vi "Complete_Controller_w_optics - Copy.vi"() -> ()   [LabVIEW 2014]
uses:
  <vilib>/LabVIEW Interface for Arduino/Type Defs/Arduino Resource.ctl
  <vilib>/LabVIEW Interface for Arduino/Type Defs/Board Type.ctl
  <vilib>/Instr/_visa.llb/VISA Configure Serial Port (Instr).vi
  <vilib>/Utility/file.llb/Write To Spreadsheet File (string).vi
  <vilib>/Utility/file.llb/Write To Spreadsheet File (DBL).vi
  <vilib>/Utility/file.llb/Read From Spreadsheet File (string).vi
  <vilib>/DAQmx/read.llb/DAQmx Read (Analog 1D DBL NChan 1Samp).vi
  <vilib>/DAQmx/write.llb/DAQmx Write (Analog 1D DBL NChan 1Samp).vi
  <vilib>/DAQmx/write.llb/DAQmx Write (Digital Bool 1Line 1Point).vi
  Environmental Chamber LabVIEW and Instruments/Drivers and Software/keithley_6430/Keithley 6430/Public/Data/Read (Single Point).vi
  Environmental Chamber LabVIEW and Instruments/Drivers and Software/LabVIEW 8.2 Drivers/keithley_24xx/Keithley 24XX/Public/Data/Read (Single Point).vi
  Environmental Chamber LabVIEW and Instruments/Drivers and Software/keithley_24xx/Keithley 24XX/Keithley 24XX.lvlib
  Environmental Chamber LabVIEW and Instruments/Drivers and Software/keithley_6430/Keithley 6430/Keithley 6430.lvlib
  <vilib>/LabVIEW Interface for Arduino/LabVIEW Interface for Arduino.lvlib
panel:
  out "Currently saving data":bool
  in  "Data saving":T1(radio)
  in  "Integration Time (ms)":i32=80 caption="Inter scan delay ms"
  in  "Optical Smoothing Level":i32 min=0 max=4 step=1
  in  "Number of Scans to Average":i32=1 min=1 max=10000 step=1
  in  "Digitizer Clock Rate Setting":i32=3 min=1 max=3
  out "Critical Error":bool
  in  "Save spectra file path":path=path "C:/Users/User/Desktop/Chamber Data/perovskites/2015-08-04 spectra"
  in  "Aquire spectra":bool
  in  "Seconds between  spectra":dbl caption="Time Target (s)"
  out "Spectrum":cluster{"Wavelengths":dbl[], "buffer out":sgl[]}(graph)
  out "output param":i32
  out "Sequence time left (hrs)":dbl caption="min"
  out "Sequence Preview":cluster{dbl[], dbl[]}[](graph)
  out "Pressure Control 3":bool caption="Pressure Control"
  in  "valve % open":dbl=100.0 min=0.0 max=100.0 step=5.0
  in  "Vapor\nflow\n(sccm)":sgl(slide) min=0 max=100 step=1 scale=0.0..200.0
  out "Actual":dbl
  out "Boolean 3":bool
  out "Actual":dbl
  out "Boolean":bool
  in  "Gas\nflow\n(sccm)":sgl(slide) min=0 max=100 step=1 scale=0.0..200.0
  in  "Desired pressure":dbl min=0.0 max=760.0 step=5.0
  out "Valve position (%)":dbl
  in  "Pressure Control":enum32{"Set % open ", " Set pressure  (Torr)"}(radio)
  out "Pressure Control 2":bool caption="Pressure Control"
  out "Keithley 6430":bool
  out "J-Kem":bool caption="J-Kem Temp"
  out "J-Kem Temp (C)":cluster{dbl}(graph)
  out "Keithley 2420":bool caption="Keithley 2430"
  out "Pressure Control":bool
  out "SRS QCM":bool
  out "MHz":dbl format="%.6f"
  out "Ohm":dbl format="%.4e"
  out "Waveform Chart 7":cluster{dbl, "Resistance out":dbl}(graph)
  out "Chamber Pressure (Torr)":cluster{"f":dbl}(graph)
  in  "Start recording after":dbl caption="min"
  in  "Auto stop after":bool
  in  "hrs":dbl=1000.0 min=0.0
  out "Start Time":string
  out "Elapsed (min)":dbl caption="Elapsed Time (s)"
  in  "Delay between data points (s)":dbl caption="sec" min=0.0 max=30.0 format="%#_13g"
  in  "Turbo pump auto on":bool=TRUE
  in  "stop":bool
  in  "Experiment Notes":string
  in  "Clear all charts":bool
  out "Save data file path":path
  out "Waveform Chart 2":cluster{"f":dbl, "f":dbl}(graph)
  out "Keithley 2420 (Ohm)":cluster{"Resistance":sgl}(graph)
  out "Keithley 6430 (Ohm)":cluster{"Measurement":dbl}(graph)
  in  "Tab Control":T2(tab)
  out "run sequence table":string[][](table) caption="Sequence to run"
  in  "Run Sequence":bool
  out "Current step":i32
  out "Step time remaining (min)":dbl caption="min" format="%#_1g"
  in  "Import sequence file":path
  in  "Use excel file\nfor sequence?":bool
  in  "Pressure Mode":T3(radio)
  in  "User-defined\nsequence":string[][](table) caption="Create sequence"
  in  "Partial pressure of solvent (%)":dbl=100.0 min=0.0 max=100.0 step=5.0
  in  "Arduino":bool
  out "temp\n(C)":string
  out "gas\nsensor":string
  out "Arduino humidity (%)":cluster{dbl}(graph)
  in  "rapidox O2 Sensor":bool
  in  "setnag O2 Pump":bool
  in  "Baud Rate 2":i32(ring)=2 items=["2400", "4800", "9600", "19200", "38400", "57600", "115200"]
  in  "Com Port":i32(ring) items=["Com 1", "Com 2", "Com 3", "Com 4", "Com 5", "Com 6", "COM 7", "COM 8", "COM 9", "COM 10", "COM 11", "COM 12", "com 13", "COM 14"]
  in  "Com Port 2":i32(ring) items=["Com 1", "Com 2", "Com 3", "Com 4", "Com 5", "Com 6", "COM 7", "COM 8", "COM 9", "COM 10", "COM 11", "COM 12", "com 13", "COM 14"]
  out "Torr":dbl
  out "%":dbl
  out "atm":dbl
  out "Waveform Chart":cluster{dbl}(graph)
  out "O2 Concentration (PPM)":dbl
  out "Waveform Chart 6":cluster{dbl}(graph)
  out "Waveform Chart 8":cluster{dbl, "Resistance out":dbl}(graph)
  # "QCM"
  # "Currently Unused"
  # "QCM"
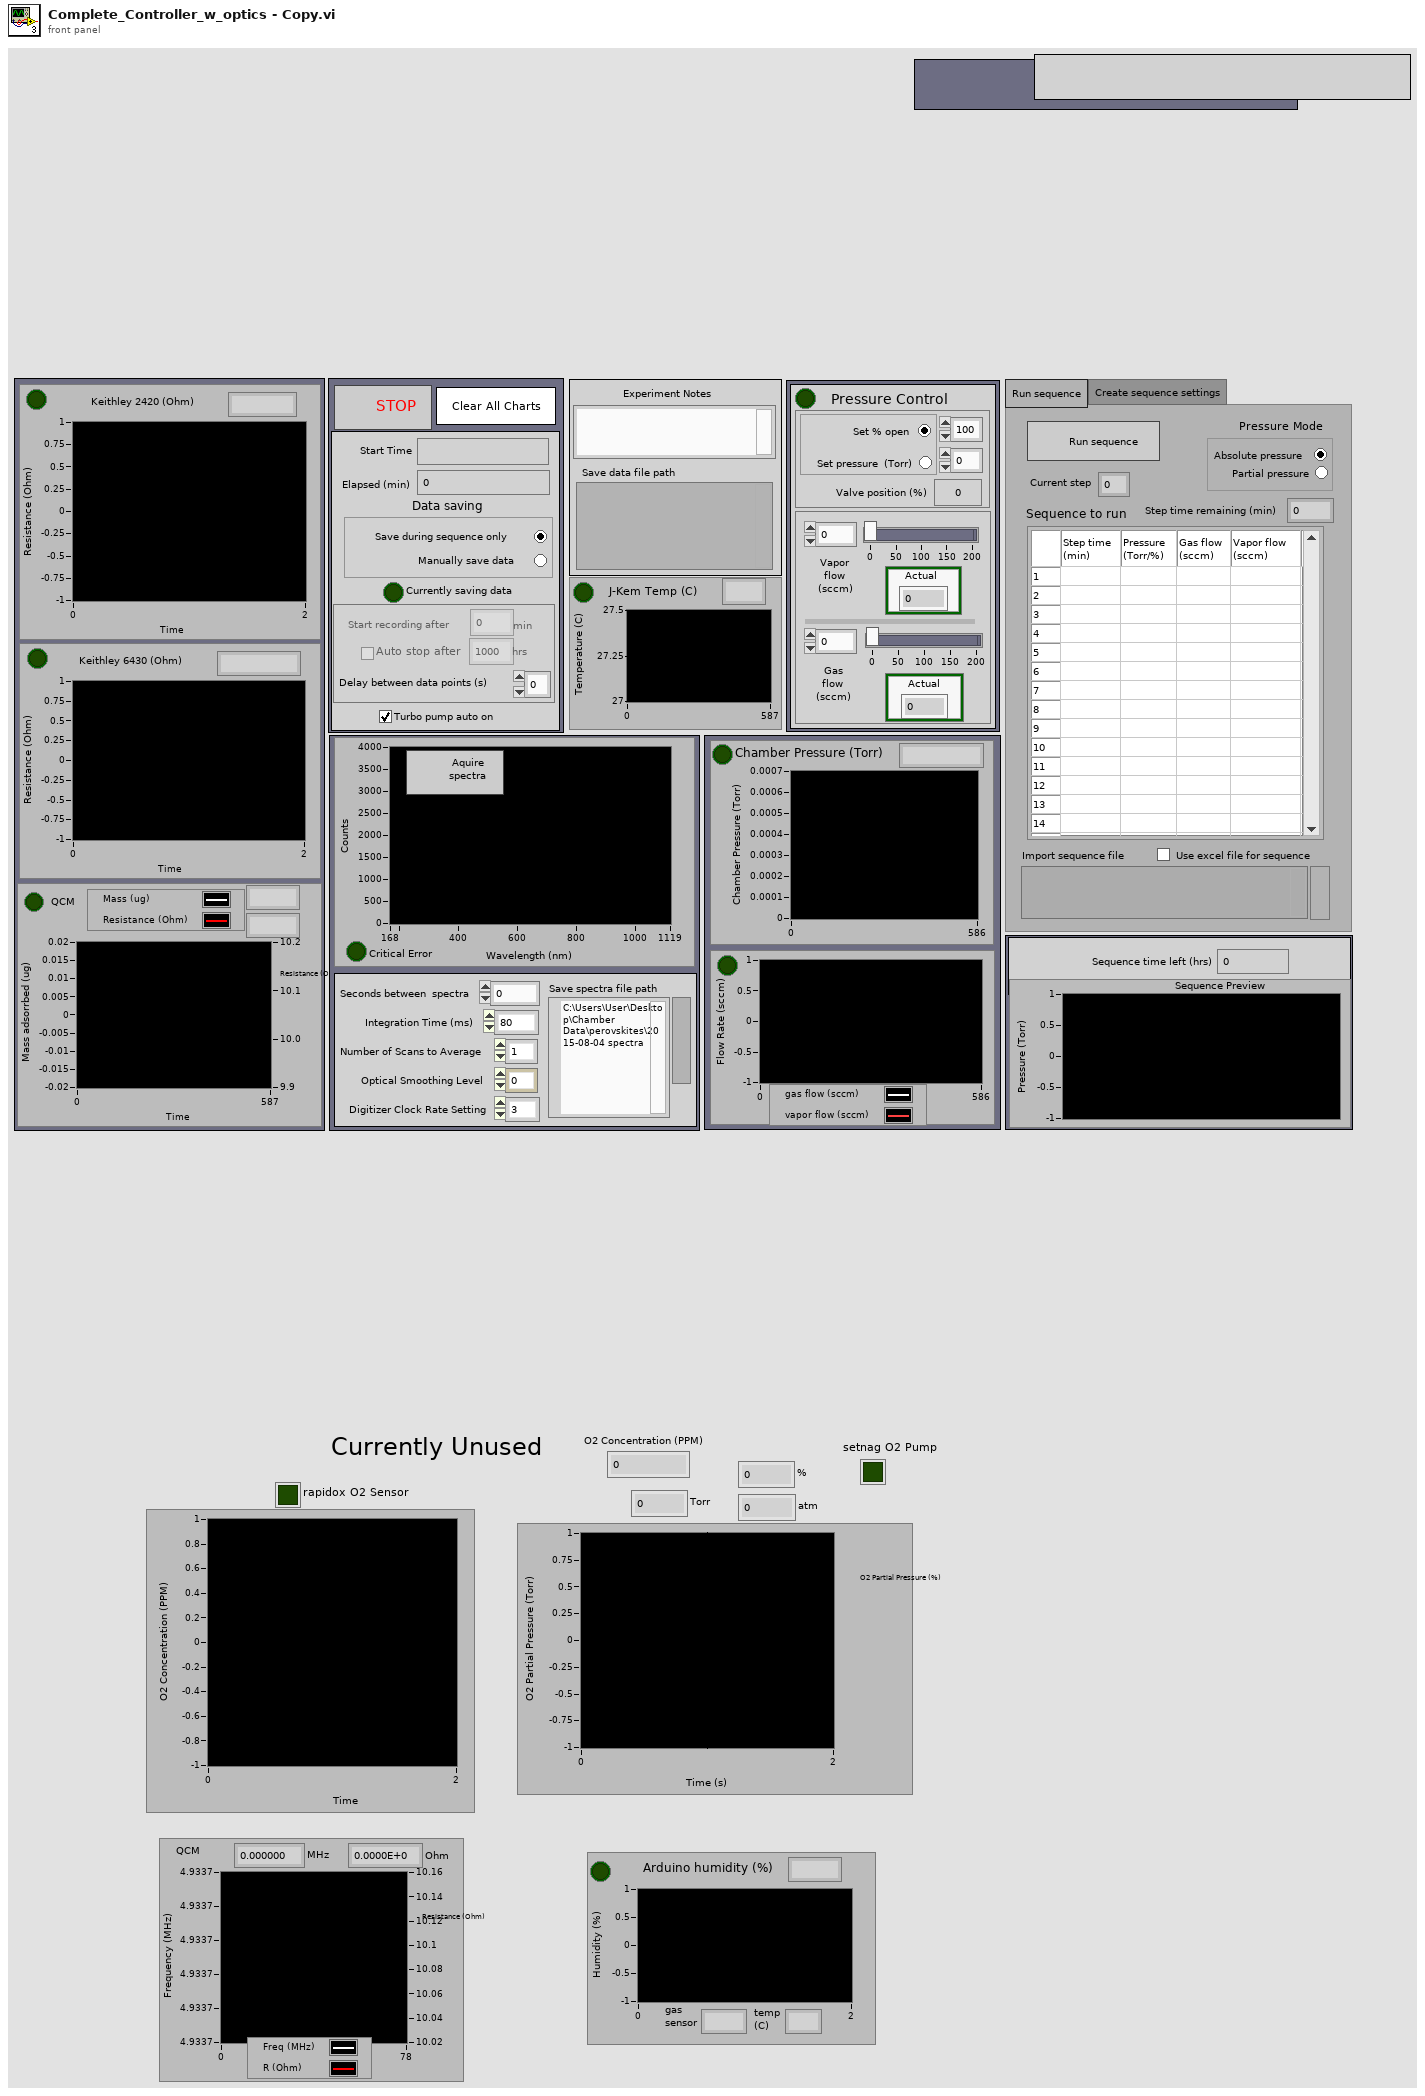
[diagram p1: front panel]
types:
  T1 = enum32{"Save during sequence only", " Manually save data"}
  T2 = enum32{"Run sequence", "Create sequence settings"}
  T3 = enum32{"Absolute pressure ", " Partial pressure"}
  T4 = enum16{"open", "open or create", "create or replace", "create", "open (read only)"}
  T5 = enum16{"no parity", "odd parity", "even parity", "mark parity", "space parity"}
  T6 = cluster{bool, "VISA resource name":refnum<visa-resource-name>, "error out":errorcluster}
  T7 = cluster{bool, "VISA resource name out":refnum<visa-resource-name>, "error out":errorcluster}
  T8 = cluster{"task out":refnum<k21>, "error out":errorcluster, "task out":refnum<k21>, "error out":errorcluster, "task out":refnum<k21>, "error out":errorcluster, "VISA resource name":refnum<visa-resource-name>, "error out":errorcluster}
  T9 = cluster{"task out":refnum<k21>, "error out":errorcluster, "task out":refnum<k21>, "error out":errorcluster, "task out":refnum<k21>, "error out":errorcluster, "VISA resource name out":refnum<visa-resource-name>, "error out":errorcluster}
  T10 = cluster{"Coefficients":ext[], "Wavelengths":dbl[]}[]
  T11 = cluster{"Integration Time (ms)":i32, "Number of Scans to Average":i32, "Optical Smoothing Level":i32, "Digitizer Clock Rate Setting":i32, "Temp  Compensation ":bool}[]
  T12 = cluster{"Integration Time (ms)":i32, "Number of Scans to Average":i32, "Optical Smoothing Level":i32, "Digitizer Clock Rate Setting":i32, "Temp  Compensation ":bool}
  T13 = cluster{"Coefficients":ext[], "Wavelengths":dbl[]}
  T14 = cluster{bool, "VISA out":refnum<visa-resource-name>, "error out":errorcluster}
  T15 = cluster{"Boolean":bool, "VISA resource name out":refnum<visa-resource-name>, "error out":errorcluster}
  T16 = enum8{"Enabled", "Disabled", "Disabled and Grayed Out"}
  T17 = typedef "LabVIEW Interface for Arduino.lvlib/Arduino Resource.ctl" = cluster{"VISA resource":refnum<visa-resource-name>, "Board Type":T18, "Connection Type":enum8{"USB / Serial"}, "Bytes Per Packet (15)":u8}
  T18 = typedef "LabVIEW Interface for Arduino.lvlib/Board Type.ctl" = enum16{"Uno", "Dimuelanove w/Atmega 328", "Mega 2560"}
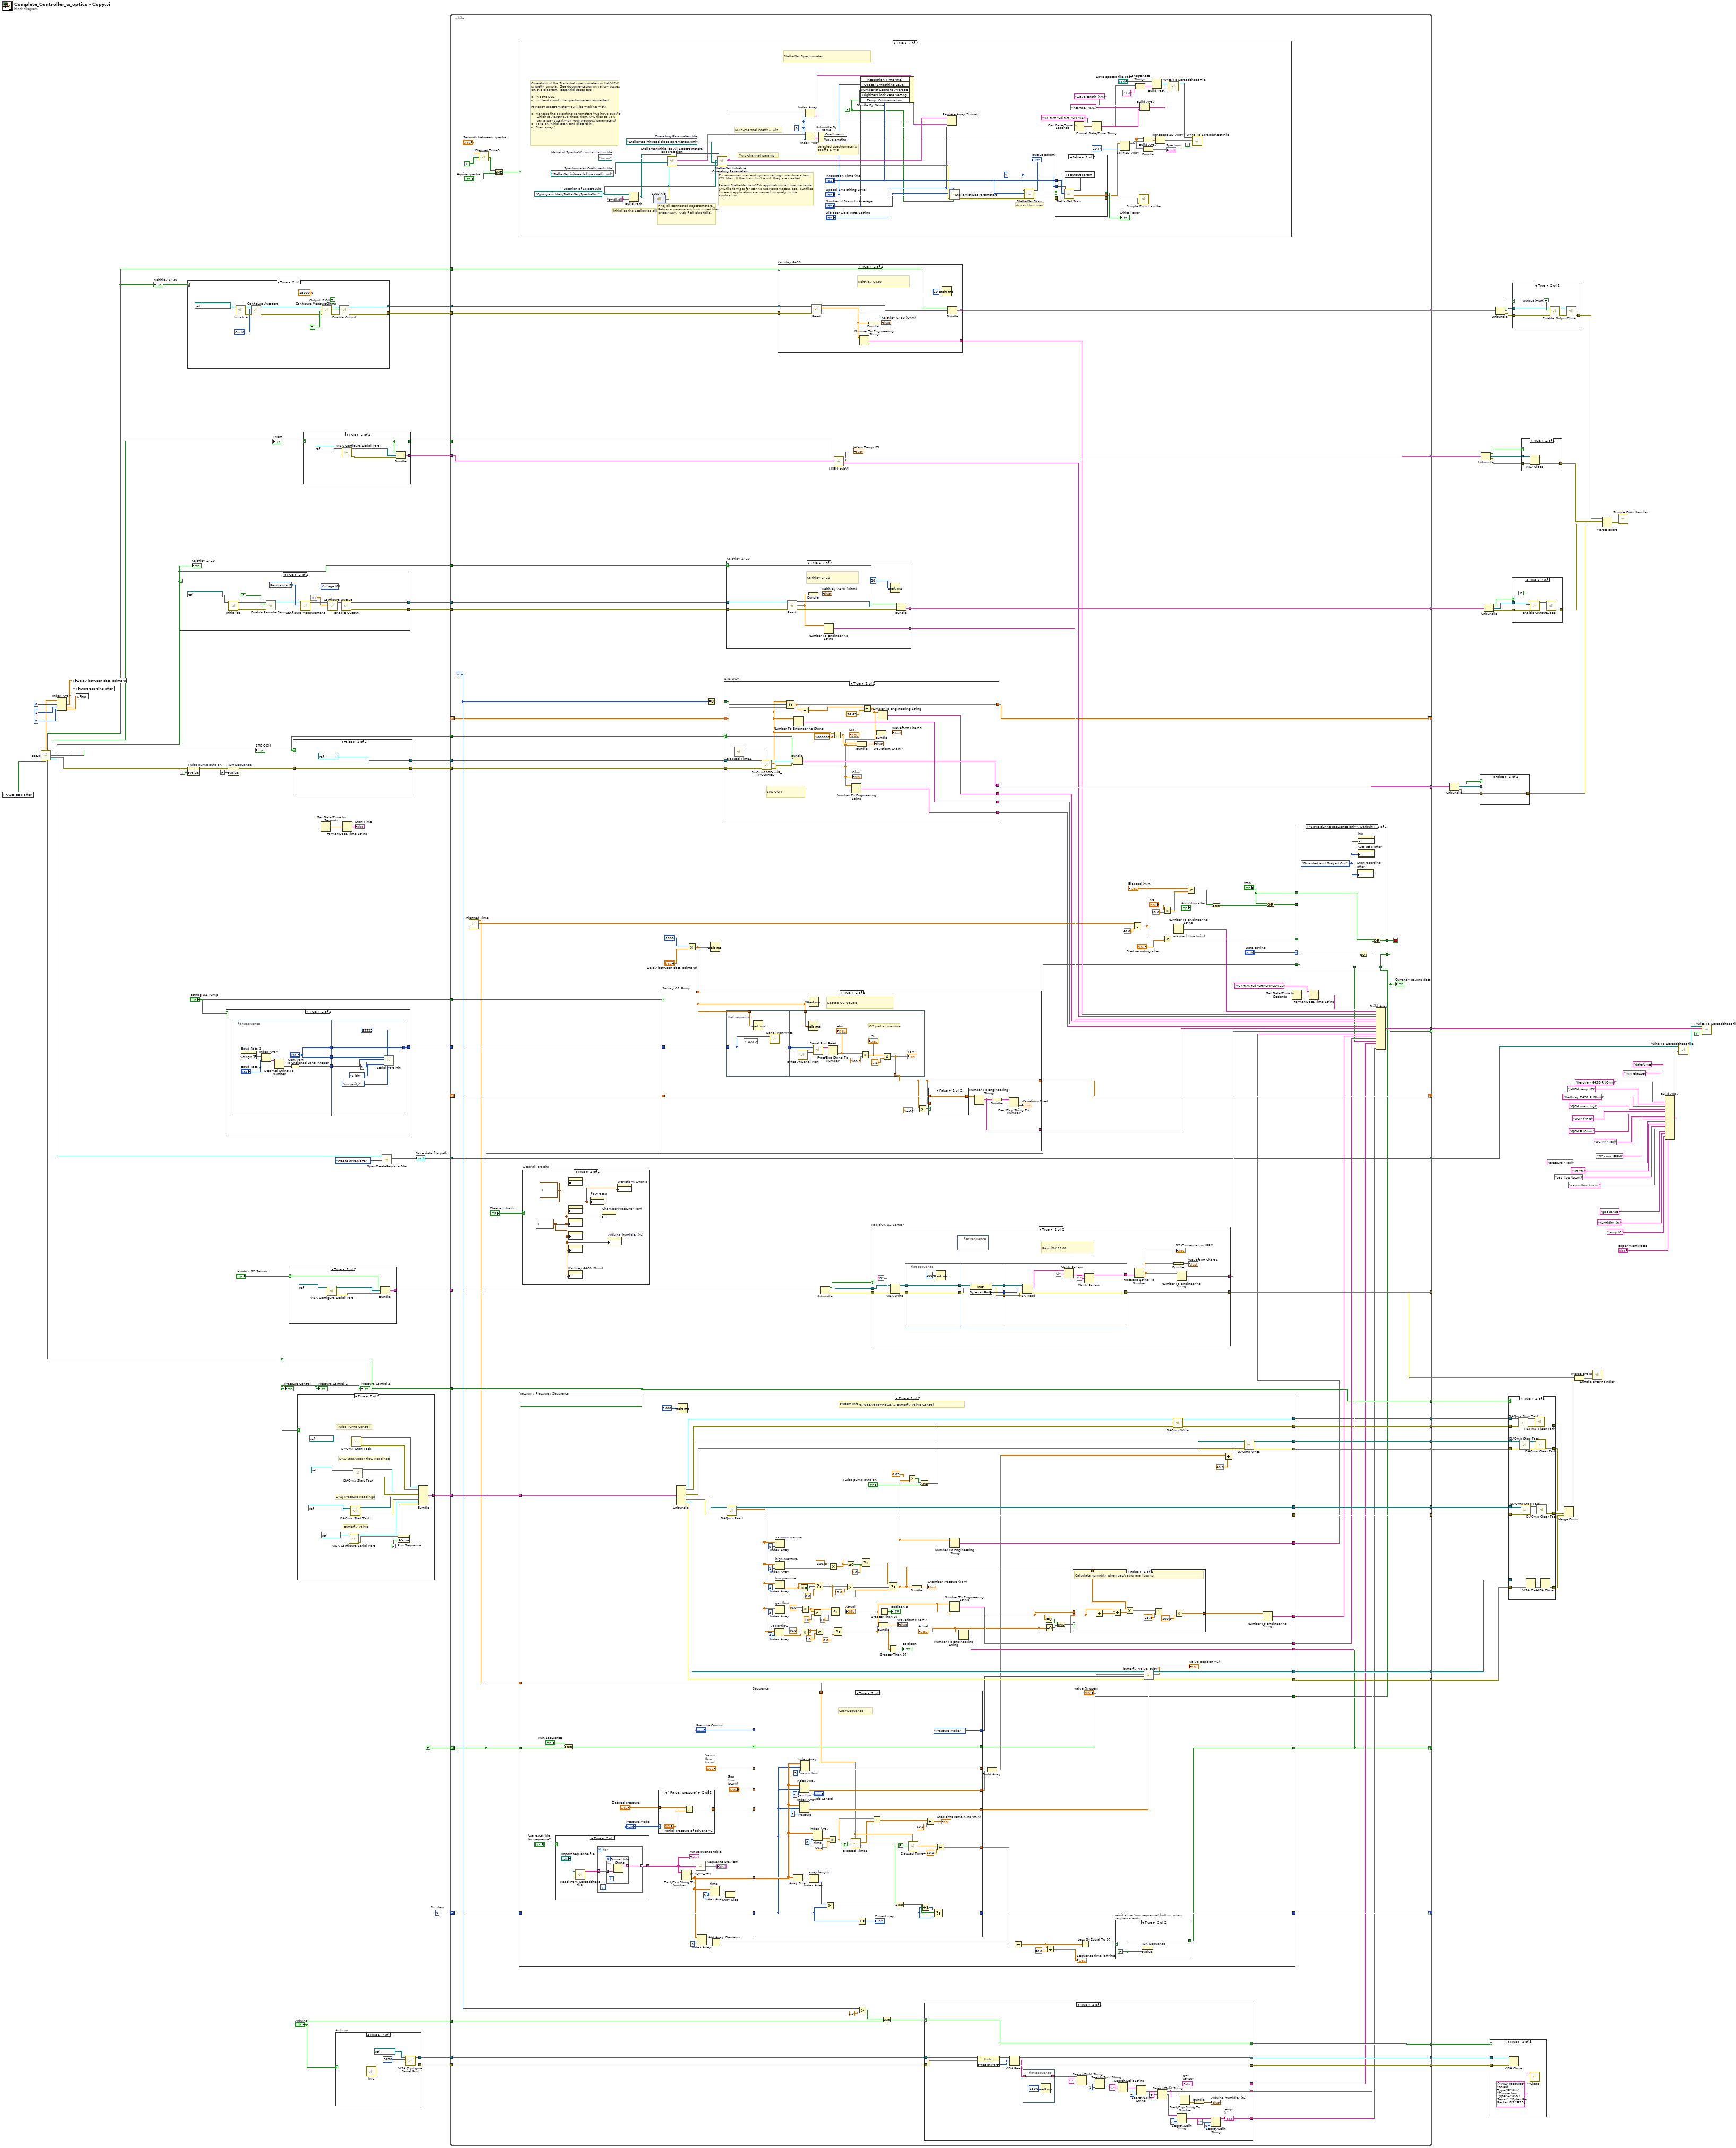
[diagram p0: block diagram]
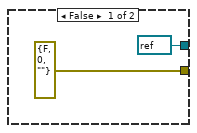
[diagram p3: hidden frame]
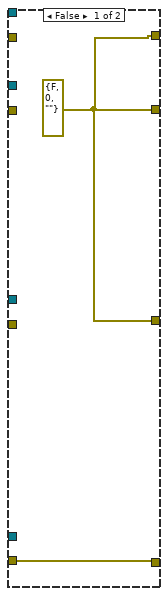
[diagram p4: hidden frame]
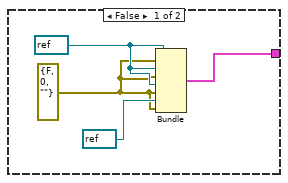
[diagram p5: hidden frame]
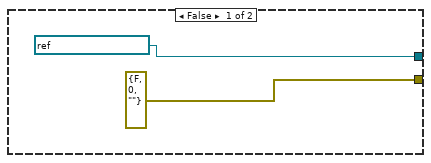
[diagram p7: hidden frame]
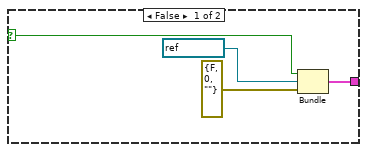
[diagram p8: hidden frame]
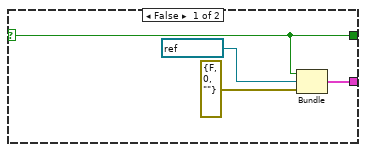
[diagram p10: hidden frame]
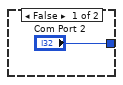
[diagram p11: hidden frame]
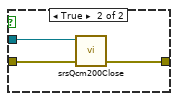
[diagram p12: hidden frame]
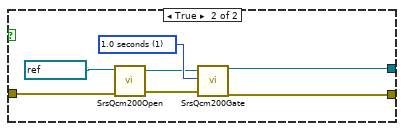
[diagram p13: hidden frame]
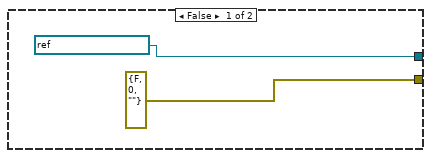
[diagram p15: hidden frame]
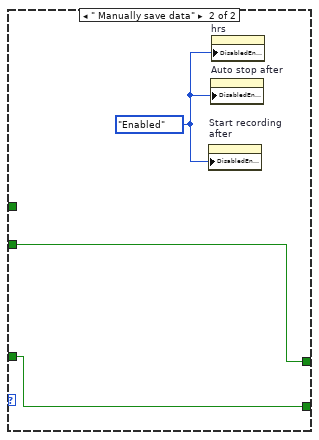
[diagram p16: hidden frame]
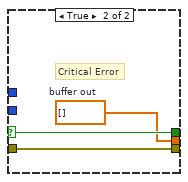
[diagram p18: hidden frame]
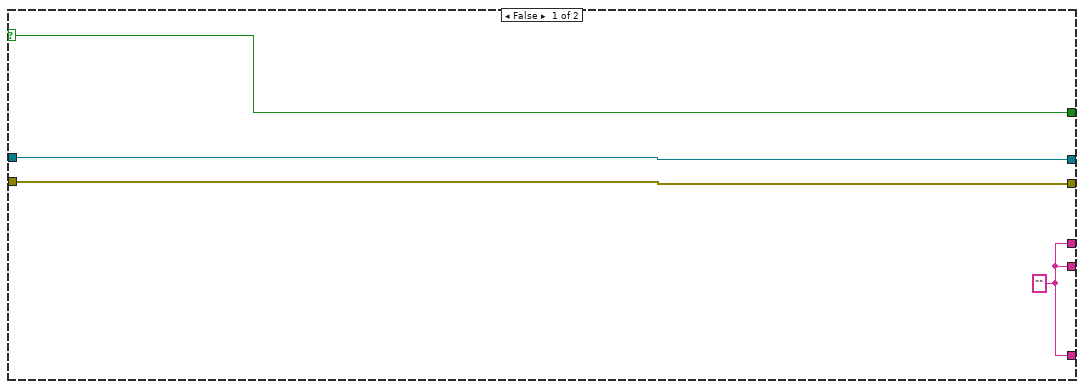
[diagram p19: hidden frame]
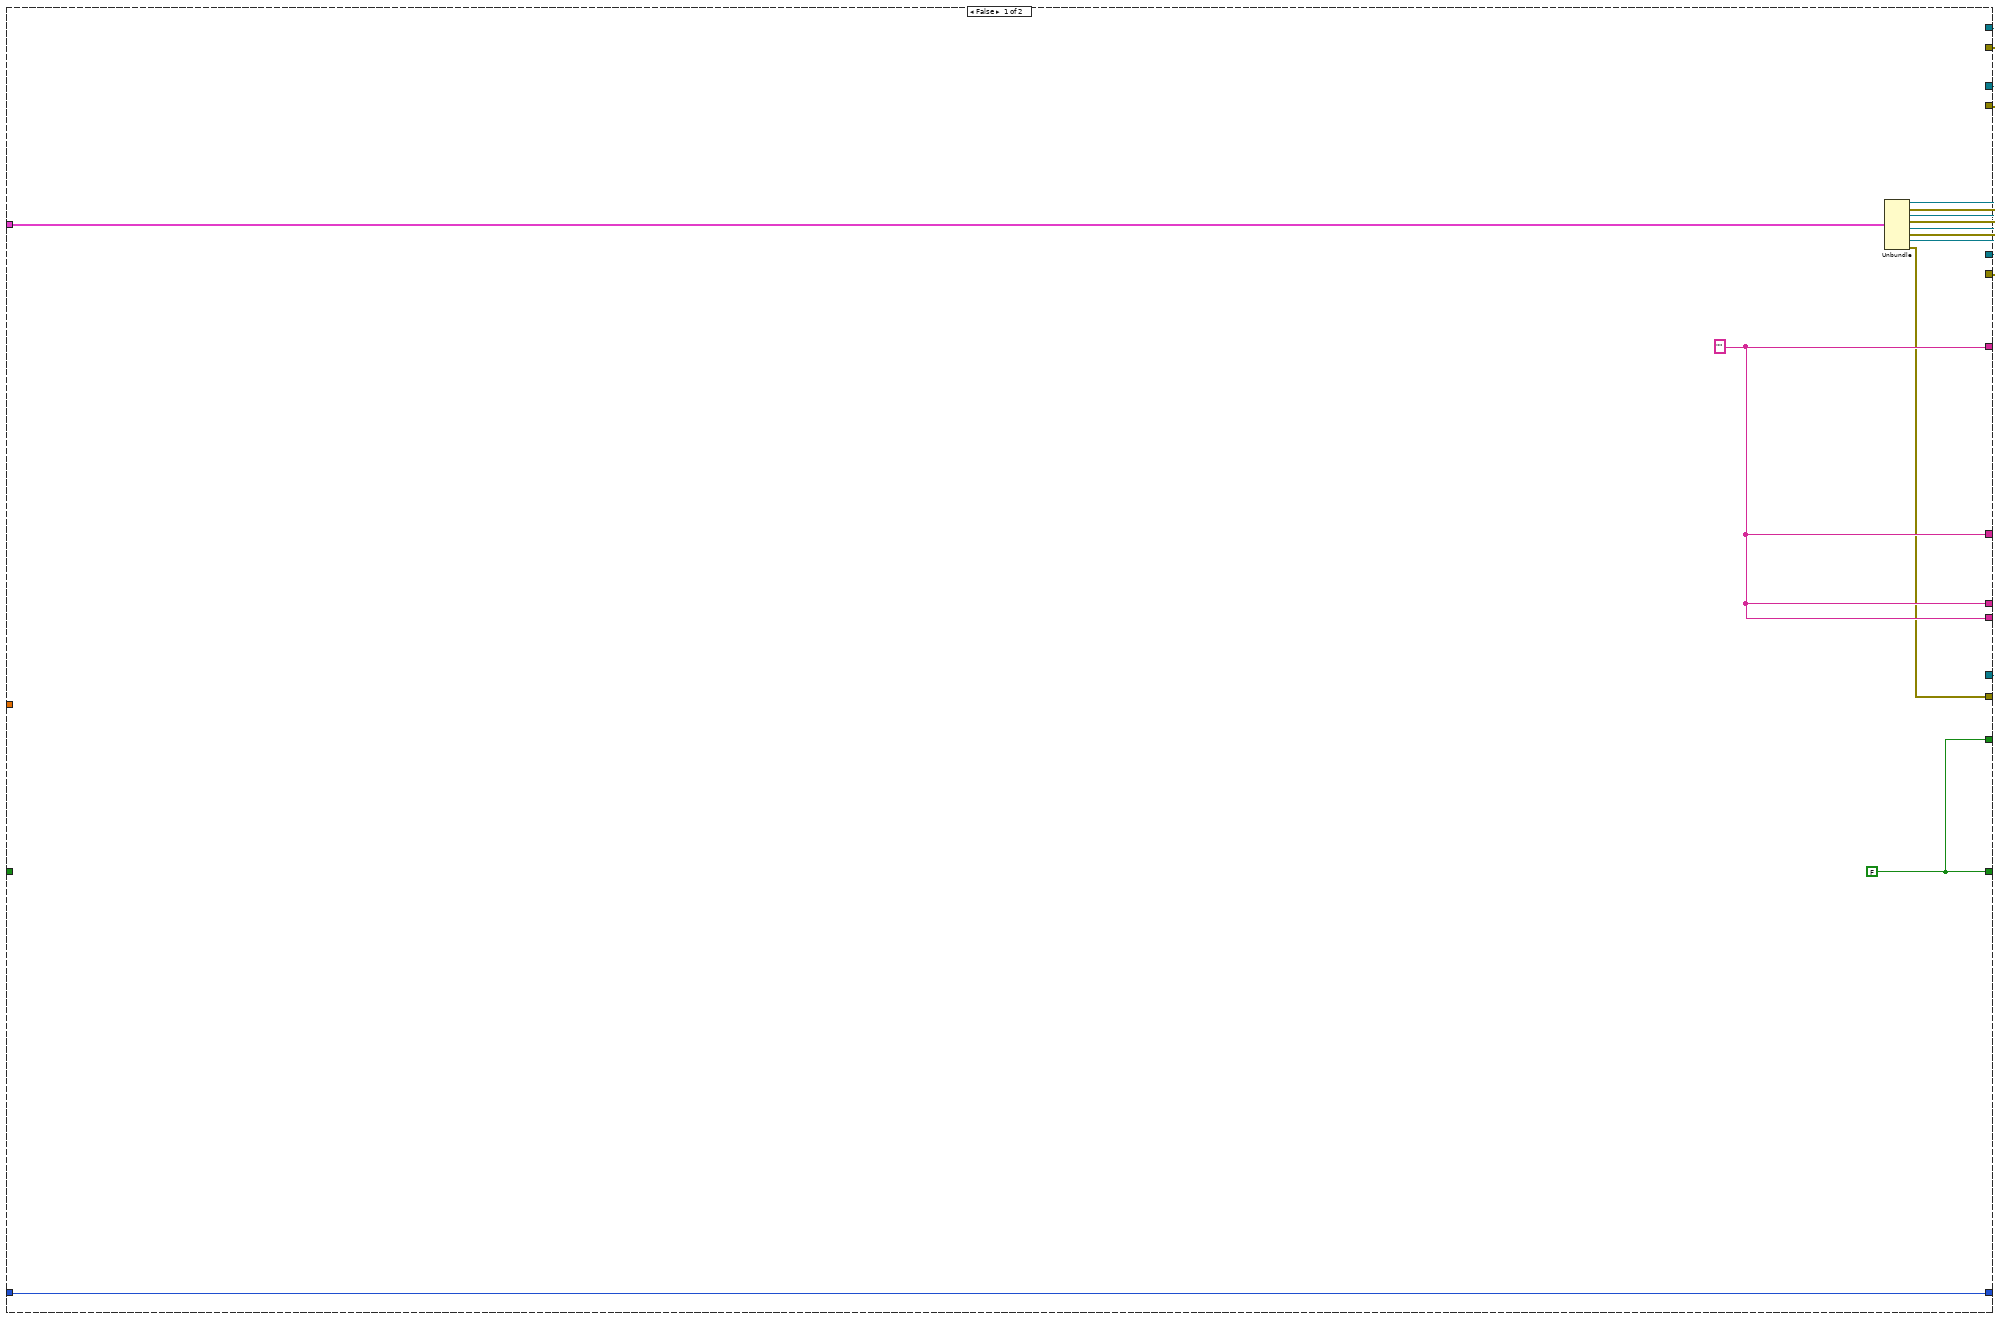
[diagram p20: hidden frame]
diagram:
  w36 = 0  # 1st step
  n1 = call "setup.vi"() -> ("delay, begin, stop settings 2"=w12:dbl[], "Keithley 6431"=w1:bool, "J-KEM2"=w2:bool, "Keithley 2421"=w6:bool, "SRS QCM 2"=w7:bool, "error IO"=w3:errorcluster, "Auto Stop 2"=w8:bool, "Pressure control 2"=w4:bool, "Save file path 2"=w5:path)  [unwired: 7 in]
  "SRS QCM" <- w7
  "Pressure Control" <- w4
  "Keithley 2420" <- w6
  "J-Kem" <- w2
  "Keithley 6430" <- w1
  "Pressure Control 2" <- w4
  "Pressure Control 3" <- w4
  n2 = local write "Auto stop after"(w8) -> ()
  n3 = Index Array(array=w12, index #1=0 ("index"), index #2=1 ("index"), index #3=2 ("index")) -> (element #1=w11:dbl, element #2=w10:dbl, element #3=w9:dbl)
  n4 = local write "Delay between data points (s)"(w11) -> ()
  n5 = local write "Start recording after"(w10) -> ()
  n6 = local write "hrs"(w9) -> ()
  n7 = case shown="True" w6 {
    tunnel: [refnum<visa-resource-name> "GPIB1::24::INSTR" ("VISA resource name") w113] -> w101
    tunnel: [errorcluster {"status"=FALSE, "code"=0, "source"=""} ("error out") w108] -> w100
    frame False {
    }
    frame True {
      w115 = u16 0 items=["Voltage", "Current"] ("Source Mode  (0: Voltage)")
      w120 = u16 2 items=["Volts", "Current", "Resistance"] ("Function (0: Volts)")
      n8 = call "Initialize.vi"("VISA resource name"=refnum<visa-resource-name> "GPIB1::24::INSTR") -> ("error out"=w109:errorcluster, "VISA resource name out"=w112:refnum<visa-resource-name>)  [unwired: 9 in]
      n9 = call "Enable Remote Sensing.vi"("error in (no error)"=w109, "Enable Remote Sensing (T: Enable)"=FALSE ("4-wire?"), "VISA resource name"=w112) -> ("error out"=w110:errorcluster, "VISA resource name out"=w111:refnum<visa-resource-name>)  [unwired: 7 in]
      n10 = call "Configure Measurement.vi"("error in (no error)"=w110, "Function (0: Volts)"=w120, "VISA resource name"=w111) -> ("error out"=w119:errorcluster, "VISA resource name out"=w118:refnum<visa-resource-name>)  [unwired: 7 in]
      n11 = call "Configure Output.vi"("Source Mode  (0: Voltage)"=w115, "error in (no error)"=w119, "Output Level (0)"=0.1 ("Applied Voltage (V)"), "VISA resource name"=w118) -> ("error out"=w117:errorcluster, "VISA resource name out"=w116:refnum<visa-resource-name>)  [unwired: 6 in]
      n12 = call "Enable Output.vi"("error in (no error)"=w117, "VISA resource name"=w116) -> ("error out"=w108:errorcluster, "VISA resource name out"=w113:refnum<visa-resource-name>)  [unwired: 8 in]
    }
  }
  n13 = case shown="True" w1 {
    tunnel: [refnum<visa-resource-name> "GPIB0::29::INSTR" ("VISA resource name") w130] -> w59
    tunnel: [errorcluster {"status"=FALSE, "code"=0, "source"=""} ("error out") w131] -> w58
    frame False {
    }
    frame True {
      (unwired) 15000.0 ("Resistance Range [Ohms]")
      w126 = u16 0 items=["On", "Off", "Once"] ("Autozero  (0: On)")
      w134 = TRUE  # Output (F:Off)
      n14 = call "Initialize.vi"("VISA resource name"=refnum<visa-resource-name> "GPIB0::29::INSTR") -> ("error out"=w127:errorcluster, "VISA resource name out"=w128:refnum<visa-resource-name>)  [unwired: 4 in, 5 out]
      n15 = call "Configure Autozero.vi"("error in (no error)"=w127, "Autozero  (0: On)"=w126, "VISA resource name"=w128) -> ("error out"=w124:errorcluster, "VISA resource name out"=w125:refnum<visa-resource-name>)  [unwired: 7 in]
      n16 = call "Configure MeasureOhms.vi"("error in (no error)"=w124, "Auto Range (T:Enable)"=TRUE, "VISA resource name"=w125) -> ("error out"=w135:errorcluster, "VISA resource name out"=w133:refnum<visa-resource-name>)  [unwired: 3 in, 4 out]
      n17 = call "Enable Output.vi"("error in (no error)"=w135, "Enable Output (F:Off)"=w134, "VISA resource name"=w133) -> ("error out"=w131:errorcluster, "VISA resource name out"=w130:refnum<visa-resource-name>)  [unwired: 7 out]
    }
  }
  n18 = property on="Turbo pump auto on" class="Bool (strict)"(error in=w3, "Value"=TRUE ("Turbo\npump")) -> (error out=w21:errorcluster)  [unwired: 1 in, 1 out]
  n19 = case shown="True" "setnag O2 Pump" {
    tunnel: ["Com Port 2" w137] -> w97
    frame False {
    }
    frame True {
      n20 = flat-sequence {
        tunnel: ["Com Port"] -> w140
        tunnel: [w142] -> w139
        tunnel: ["Com Port"] -> w138
        tunnel: w140 -> [w148]
        tunnel: w139 -> [w147]
        tunnel: w138 -> [w149]
        tunnel: [w149] -> w137
        frame #0 {
          n21 = property on="Baud Rate 2" class="Ring (strict)"() -> ("Strings []"=w144:string[])  [unwired: 2 in, 2 out]
          n22 = Index Array(array=w144, index="Baud Rate 2") -> (element=w145:string)
          n23 = Decimal String To Number(string=w145) -> (number=w143:i32)  [unwired: 2 in, 1 out]
          n24 = To Unsigned Long Integer(number=w143) -> (unsigned 32bit integer=w142:u32)
        }
        frame #1 {
          n25 = call <vilib>:"Serial Port Init.vi"("parity"=T5."no parity", "buffer size"=u16 65535, "stop bits"=enum16{"1 bit", "1.5 bits", "2 bits"}."1 bit", "data bits"=u16 8, "baud rate"=w147, "port number"=w148) -> ()  [unwired: 1 in, 1 out]
        }
      }
    }
  }
  n26 = property on="Run Sequence" class="Bool (strict)"(error in=w21, "Value"=FALSE ("Run Sequence")) -> (error out=w25:errorcluster)  [unwired: 1 in, 1 out]
  n27 = case shown="True" "rapidox O2 Sensor" {
    selector: "rapidox O2 Sensor" -> [w154 w159]
    tunnel: [w155 w160] -> w68
    frame False {
      n28 = Bundle(w154, "VISA resource name"=refnum<visa-resource-name> "COM7", "error out"=errorcluster {"status"=FALSE, "code"=0, "source"=""}) -> (w155:T6)  [unwired: 1 in]
    }
    frame True {
      n29 = call-poly "VISA Configure Serial Port"("VISA resource name"=refnum<visa-resource-name> "COM7") -> ("VISA resource name out"=w161:refnum<visa-resource-name>, "error out"=w158:errorcluster)  [unwired: 13 in]
      n30 = Bundle(w159, "VISA resource name out"=w161, "error out"=w158) -> (w160:T7)  [unwired: 1 in]
    }
  }
  n31 = case shown="False" w7 {
    tunnel: [refnum<visa-resource-name> "COM6" ("VISA in") w167] -> w99
    tunnel: [w163 w166] -> w98
    tunnel: w25 -> [w163 w165]
    frame False {
    }
    frame True {
      w171 = u16 1 items=["0.1 seconds", "1.0 seconds", "10.0 seconds"] ("Gate in")
      n32 = call "SrsQcm200Open.vi"("error in"=w165, "VISA in"=refnum<visa-resource-name> "COM6") -> ("error out"=w168:errorcluster, "VISA out"=w169:refnum<visa-resource-name>)  [unwired: 3 in]
      n33 = call "SrsQcm200Gate.vi"("VISA in"=w169, "Gate in"=w171, "error in (no error)"=w168) -> ("VISA out"=w167:refnum<visa-resource-name>, "error out"=w166:errorcluster)  [unwired: 14 in, 1 out]
    }
  }
  n34 = case shown="True" w4 {
    tunnel: [w172 w179] -> w41
    frame False {
      w174 = refnum<k21> refnum ("task out")
      w173 = errorcluster {"status"=FALSE, "code"=0, "source"=""} ("error out")
      n35 = Bundle("task out"=w174, "error out"=w173, "task out"=w174, "error out"=w173, "task out"=w174, "error out"=w173, "VISA resource name"=refnum<visa-resource-name> refnum, "error out"=w173) -> (w172:T8)  [unwired: 1 in]
    }
    frame True {
      # "Turbo Pump Control"
      # "DAQ Gas/Vapor Flow Readings"
      # "DAQ Pressure Readings"
      # "Butterfly Valve"
      n36 = call-poly "VISA Configure Serial Port"("VISA resource name"=refnum<visa-resource-name> "COM5") -> ("VISA resource name out"=w180:refnum<visa-resource-name>, "error out"=w176:errorcluster)  [unwired: 13 in]
      n37 = call <vilib>:"DAQmx Start Task.vi"("task/channels in"=refnum<k21> "AllDaqReadings") -> ("task out"=w182:refnum<k21>, "error out"=w181:errorcluster)  [unwired: 13 in]
      n38 = call <vilib>:"DAQmx Start Task.vi"("task/channels in"=refnum<k21> "TurboON") -> ("task out"=w186:refnum<k21>, "error out"=w185:errorcluster)  [unwired: 13 in]
      n39 = call <vilib>:"DAQmx Start Task.vi"("task/channels in"=refnum<k21> "Setflow") -> ("task out"=w184:refnum<k21>, "error out"=w183:errorcluster)  [unwired: 13 in]
      n40 = property on="Run Sequence" class="Bool (strict)"(error in=w176, "Value"=FALSE ("Run Sequence")) -> (error out=w178:errorcluster)  [unwired: 1 in, 1 out]
      n41 = Bundle("task out"=w186, "error out"=w185, "task out"=w184, "error out"=w183, "task out"=w182, "error out"=w181, "VISA resource name out"=w180, "error out"=w178) -> (w179:T9)  [unwired: 1 in]
    }
  }
  n42 = case shown="True" w2 {
    selector: w2 -> [w191 w196]
    tunnel: [w192 w197] -> w86
    tunnel: [w191 w196] -> w80
    frame False {
      n43 = Bundle(w191, "VISA resource name"=refnum<visa-resource-name> "COM3", "error out"=errorcluster {"status"=FALSE, "code"=0, "source"=""}) -> (w192:T6)  [unwired: 1 in]
    }
    frame True {
      n44 = call-poly "VISA Configure Serial Port"("VISA resource name"=refnum<visa-resource-name> "COM3") -> ("VISA resource name out"=w198:refnum<visa-resource-name>, "error out"=w195:errorcluster)  [unwired: 13 in]
      n45 = Bundle(w196, "VISA resource name out"=w198, "error out"=w195) -> (w197:T7)  [unwired: 1 in]
    }
  }
  n46 = Get Date/Time In Seconds() -> (seconds since 1Jan1904=w104:timestamp)
  n47 = case "Arduino" shown="True" "Arduino" {
    tunnel: [refnum<visa-resource-name> refnum ("VISA resource name out") w205] -> w35
    tunnel: [errorcluster {"status"=FALSE, "code"=0, "source"=""} ("error out") w202] -> w34
    frame False {
    }
    frame True {
      n48 = call <vilib>:"Init.vi"() -> ()  [unwired: 18 in, 2 out]
      n49 = call-poly "VISA Configure Serial Port"("VISA resource name"=refnum<visa-resource-name> "COM12", "baud rate (9600)"=u32 9600) -> ("VISA resource name out"=w205:refnum<visa-resource-name>, "error out"=w202:errorcluster)  [unwired: 12 in]
    }
  }
  n50 = Format Date/Time String(seconds (now)=w104) -> (date/time string=→"Start Time":string)  [unwired: 2 in]
  n51 = call "OpenCreateReplace File.vi"("function (open:0)"=T4."create or replace", "file path"=w5) -> ("new file path"=w27:path)  [unwired: 6 in, 3 out]
  "Save data file path" <- w27
  n52 = while {
    shift-right: [w303] -> _
    shift-left: _ -> [w302]
    tunnel: [w240] -> w102 mode=indexing if=w206
    tunnel: w6 -> [w272]
    tunnel: w101 -> [w300]
    tunnel: w100 -> [w299]
    tunnel: w99 -> [w298]
    tunnel: w98 -> [w297]
    tunnel: w7 -> [w295]
    tunnel: "setnag O2 Pump" -> [w288]
    tunnel: w97 -> [w294]
    tunnel: [w290] -> w94
    tunnel: [w289] -> w90
    tunnel: w86 -> [w287]
    tunnel: [w286] -> w85
    tunnel: w80 -> [w284]
    tunnel: w68 -> [w281]
    tunnel: [w276] -> w17
    tunnel: [w271] -> w66
    tunnel: w27 -> [w271]
    shift-right: [w217] -> _
    shift-left: _ -> [w218]
    tunnel: w59 -> [w269]
    tunnel: w58 -> [w268]
    tunnel: [w267] -> w57
    tunnel: w1 -> [w266]
    tunnel: w4 -> [w252]
    tunnel: [w264] -> w53
    tunnel: [w263] -> w50
    tunnel: [w262] -> w52
    tunnel: [w261] -> w51
    tunnel: [w252] -> w49
    tunnel: [w260] -> w45
    tunnel: w41 -> [w256]
    tunnel: [w255] -> w39
    tunnel: [w254] -> w38
    tunnel: [w253] -> w37
    shift-right: [w251] -> _
    shift-left: w36 -> [w250]
    tunnel: "Arduino" -> [w237]
    tunnel: w35 -> [w246]
    tunnel: w34 -> [w245]
    tunnel: [w244] -> w33
    tunnel: [w243] -> w32
    tunnel: [w242] -> w31
    shift-right: [w208] -> _
    shift-left: TRUE -> [w207]
    i -> [w229]
    stop <- w214 stop-if-true
    n53 = call "Elapsed Time"() -> ("Present (s)"=w249:dbl, "Elapsed Time (s)"=w283:dbl)  [unwired: 12 in, 6 out]
    n54 = call "Elapsed Time5"("Time Target (s)"="Seconds between  spectra", "Auto Reset"=TRUE) -> ("Time has Elapsed"=w223:bool)  [unwired: 10 in, 7 out]
    n55 = And(x=w223, y="Aquire spectra") -> (x .and. y?=w221:bool)
    n56 = case shown="True" w221 {
      frame False {
      }
      frame True {
        w329 = 0 ("Spectral Channel")
        w331 = 1 ("Spectral Channel")
        w335 = FALSE ("Temp  Compensation")
        w343 = path "C:/program files/StellarNet/SpectraWiz"  # Location of SpectraWiz
        w353 = path "sw.ini"  # Name of SpectraWiz initialization file
        w345 = path "StellarNet init-read-close parameters.xml"  # Operating Parameters file
        w354 = path "StellarNet init-read-close coeffs.xml"  # Spectrometer Coefficients file
        # "StellarNet Spectrometer"
        # "Operation of the StellarNet spectrometers in LabVIEW\nis pretty simple.  See documentation in yellow boxes\non this diagram.  Essential steps are:\n\no  init the DLL\no  init (and count) the spectrometers connected\n\nFor each spectrometer you'll be working with:\n\no  manage the operating parameters (we have subVIs\n     which save/retrieve these from XML files so you\n     can always start with your previous parameters)\no  Take an initial scan and discard it\no  Scan away!"
        # "initialize the StellarNet .dll"
        # "To remember user and system settings, we store a few \nXML files.  If the files don't exist, they are created.\n\nRecent StellarNet LabVIEW applications all use the same\nXML file formats for storing user parameters, etc., but files\nfor each application are named uniquely to the \napplication."
        # "Find all connected spectrometers.  Retrieve parameters from stored files or EEPROM.  (Ask if all else fails)."
        # "selected spectrometer's\ncoeff's & wls"
        # "Multi-channel coeffs & wls"
        # "Multi-channel params"
        # "discard first scan"
        n57 = Build Path(base path=w343, name or relative path="swdll.dll") -> (appended path=w341:path)
        n58 = dll-call lib="C:/Program Files/StellarNet/SpectraWiz/swdll.dll" fn="SWDinit" label="init"(path in=w341) -> (error out=w342:errorcluster)  [unwired: 3 in, 1 out]
        n59 = call "StellarNet Initialize All Spectrometers, ext precision.vi"("Path of swdll.dll"=w341, "error in"=w342, "Spectrometer Coefficients file"=w354, "Location of SpectraWiz"=w343, "Name of SpectraWiz initialization file"=w353) -> ("error out"=w352:errorcluster, "Multi Channel Coeffs & WLs"=w350:T10, "Number of Channels"=w351:i32)  [unwired: 2 in, 2 out]
        n60 = call "StellarNet Initialize Operating Parameters.vi"("error in"=w352, "Spectrometer Coefficients file"=w345, "Location of SpectraWiz"=w343, "Number of Channels"=w351) -> ("error out"=w348:errorcluster, "Operating Parameters"=w346:T11)  [unwired: 6 in]
        n61 = Index Array(array=w346, index=w329) -> (element=w347:T12)
        n62 = Index Array(array=w350, index=w329) -> (element=w349:T13)
        n63 = Unbundle By Name(w349) -> ("Wavelengths"=w333:dbl[])  [unwired: 1 out]
        n64 = Bundle By Name(cluster=w347, "Integration Time (ms)"="Integration Time (ms)", "Optical Smoothing Level"="Optical Smoothing Level", "Number of Scans to Average"="Number of Scans to Average", "Digitizer Clock Rate Setting"="Digitizer Clock Rate Setting", "Temp  Compensation"=w335) -> (w338:T12)
        n65 = Replace Array Subset(array=w346, new element=w338, index=w329) -> ()  [unwired: 1 out]
        n66 = call "StellarNet Set Parameters.vi"("Temp  Compensation"=w335, "Digitizer Clock Rate Setting"="Digitizer Clock Rate Setting", "error in (no error)"=w348, "Optical Smoothing Level"="Optical Smoothing Level", "Number of Scans to Average"="Number of Scans to Average", "Integration Time (ms)"="Integration Time (ms)") -> ("error out"=w334:errorcluster)  [unwired: 5 in]
        n67 = call "StellarNet Scan.vi"("error in (no error)"=w334, "Integration Time (msec)"="Integration Time (ms)", "Spectral Channel"=w331) -> ("error out"=w359:errorcluster, "Critical Error"=w360:bool, "output param"=→"output param":i32)  [unwired: 5 in, 1 out]
        n68 = case shown="False" w360 {
          selector: w360 -> [_ w371]
          tunnel: w331 -> [w368 _]
          tunnel: [w367 w370] -> w344
          tunnel: [w365 w371] -> w357
          tunnel: w359 -> [w364 w369]
          tunnel: [w363 w369] -> w330
          tunnel: "Integration Time (ms)" -> [w362 _]
          frame False {
            n69 = call "StellarNet Scan.vi"("error in (no error)"=w364, "Integration Time (msec)"=w362, "Spectral Channel"=w368) -> ("error out"=w363:errorcluster, "buffer out"=w367:sgl[], "Critical Error"=w365:bool, "output param"=w366:i32)  [unwired: 5 in]
            n70 = local write "output param"(w366) -> ()
          }
          frame True {
            w370 = sgl[] []  # buffer out
            # "Critical Error"
          }
        }
        "Critical Error" <- w357
        n71 = Get Date/Time In Seconds() -> (seconds since 1Jan1904=w324:timestamp)
        n72 = Format Date/Time String(time format string (%c)="%Y-%m-%d %H_%M_%S", seconds (now)=w324) -> (date/time string=w319:string)  [unwired: 1 in]
        n73 = Split 1D Array(array=w344, index=2047) -> (first subarray=w332:sgl[])  [unwired: 1 out]
        n74 = Concatenate Strings(w319, ".txt") -> (w320:string)
        n75 = call <vilib>:"Simple Error Handler.vi"("error in (no error)"=w330) -> ()  [unwired: 4 in, 5 out]
        n76 = Build Array("wavelength (nm)", "intensity (a.u.)", w319) -> (w315:string[])
        n77 = Bundle("Wavelengths"=w333, w332) -> (→"Spectrum":cluster{"Wavelengths":dbl[], sgl[]})  [unwired: 1 in]
        n78 = Build Array(w333, w332) -> (w318:dbl[][])
        n79 = Build Path(base path="Save spectra file path", name or relative path=w320) -> (appended path=w322:path)
        n80 = Transpose 2D Array(2D array=w318) -> (transposed array=w317:dbl[][])
        n81 = call-poly <vilib>:"Write To Spreadsheet File.vi"("1D data"=w315, "file path (dialog if empty)"=w322) -> ("new file path (Not A Path if cancelled)"=w316:path)  [unwired: 6 in]
        n82 = call-poly <vilib>:"Write To Spreadsheet File.vi"("append to file? (new file:F)"=TRUE, "2D data"=w317, "file path (dialog if empty)"=w316) -> ()  [unwired: 5 in, 1 out]
      }
    }
    n83 = case "Vacuum / Pressure / Sequence" shown="True" w252 {
      tunnel: [w412 w521] -> w263
      tunnel: [w413 w520] -> w261
      tunnel: [w415 w501] -> w264
      tunnel: [w414 w502] -> w262
      tunnel: [w408 w492] -> w260
      tunnel: [w409 w482] -> w259
      tunnel: [w409 w481] -> w258
      tunnel: [w409 w479] -> w257
      tunnel: w256 -> [w418 w477]
      tunnel: [w417 w468] -> w255
      tunnel: [w416 w467] -> w254
      tunnel: [w411 w466] -> w253
      tunnel: w250 -> [w410 w451]
      tunnel: [w410 w463] -> w251
      tunnel: w249 -> [_ w462]
      tunnel: w207 -> [_ w443]
      tunnel: [w407 w419] -> w208
      tunnel: [w409 w439] -> w230
      tunnel: [w407 w422] -> w211
      frame False {
        w407 = FALSE ("new element/subarray")
        w409 = ""
        n84 = Unbundle(w418) -> ("task out"=w417:refnum<k21>, "error out"=w416:errorcluster, "task out"=w415:refnum<k21>, "error out"=w414:errorcluster, "task out"=w412:refnum<k21>, "error out"=w413:errorcluster, "VISA resource name out"=w411:refnum<visa-resource-name>, "error out"=w408:errorcluster)
      }
      frame True {
        # "system info"
        # "DAQ Pressure, Gas/Vapor Flows, & Butterfly Valve Control"
        n85 = case shown="True" "Use excel file\nfor sequence?" {
          tunnel: ["User-defined\nsequence" w528] -> w431
          frame False {
          }
          frame True {
            n86 = call-poly <vilib>:"Read From Spreadsheet File.vi"("file path (dialog if empty)"="Import sequence file") -> ("all rows"=w530:string[][])  [unwired: 6 in, 4 out]
            n87 = for {
              tunnel: w530 -> [w532] mode=indexing
              tunnel: [w531] -> w528 mode=indexing
              n88 = for {
                tunnel: w532 -> [w534] mode=indexing
                tunnel: [w533] -> w531 mode=indexing
                n89 = Format Into String(w534) -> (resulting string=w533:string)  [unwired: 3 in, 1 out]
              }
            }
          }
        }
        "run sequence table" <- w431
        n90 = And(x="Run Sequence", y=w443) -> (x .and. y?=w420:bool)
        n91 = case shown="\" Partial pressure\"" "Pressure Mode" {
          tunnel: [w523 w525] -> w423
          tunnel: "Desired pressure" -> [w523 w524]
          frame "Absolute pressure ", Default {
          }
          frame " Partial pressure" {
            n92 = Divide(x=w524, y="Partial pressure of solvent (%)") -> (x/y=w525:dbl)
          }
        }
        n93 = Unbundle(w477) -> ("task out"=w470:refnum<k21>, "error out"=w469:errorcluster, "task out"=w471:refnum<k21>, "error out"=w472:errorcluster, "task out"=w473:refnum<k21>, "error out"=w474:errorcluster, "VISA resource name out"=w475:refnum<visa-resource-name>, "error out"=w476:errorcluster)
        n94 = Wait (ms)(milliseconds to wait=u32 1000) -> ()  [unwired: 1 out]
        n95 = Fract/Exp String To Number(string=w431) -> (number=w442:dbl[][])  [unwired: 3 in, 1 out]
        n96 = call "plot_usr_seq.vi"("User-defined sequence"=w431) -> ("Sequence Preview"=→"Sequence Preview":cluster{dbl[], dbl[]}[])
        n97 = Index Array(array=w442, index (col)=0 ("disabled index (col)")) -> (element=w455:dbl[])  [unwired: 1 in]
        n98 = Index Array "time"(array=w442, index (row)=0 ("disabled index (col)")) -> (element=w441:dbl[])  [unwired: 1 in]
        n99 = Add Array Elements(numeric array=w455) -> (sum=w446:dbl)
        n100 = Array Size(array=w441) -> ()  [unwired: 1 out]
        n101 = call-poly <vilib>:"DAQmx Read.vi"("task/channels in"=w473, "error in"=w474) -> ("task out"=w521:refnum<k21>, "data"=w512:dbl[], "error out"=w520:errorcluster)  [unwired: 11 in]
        n102 = case "Sequence" shown="True" w420 {
          selector: w420 -> [w552 w560]
          tunnel: w462 -> [_ w574]
          tunnel: [w558 w575] -> w463
          tunnel: w451 -> [w558 w562]
          tunnel: "Vapor\nflow\n(sccm)" -> [w557 _]
          tunnel: "Gas\nflow\n(sccm)" -> [w556 _]
          tunnel: [w557 w582] -> w459
          tunnel: [w556 w581] -> w458
          tunnel: [w555 w580] -> w447
          tunnel: w423 -> [w555 _]
          tunnel: w442 -> [_ w568]
          tunnel: "Pressure Control" -> [w554 _]
          tunnel: [w554 enum32{"Open Mode", "Pressure Mode"}."Pressure Mode" ("Pressure Control")] -> w452
          tunnel: [0.0 w571] -> w445
          tunnel: [w552 w560] -> w422
          frame False {
          }
          frame True {
            # "User Sequence"
            n103 = Array Size(array=w568) -> (size(s)=w590:i32[])
            n104 = Index Array "gas flow"(array=w568, index (row)=w562, index (col)=2 ("disabled index (col)")) -> (element=w581:dbl)
            n105 = Index Array "Pressure"(array=w568, index (row)=w562, index (col)=1 ("disabled index (col)")) -> (element=w580:dbl)
            n106 = Index Array "vapor flow"(array=w568, index (row)=w562, index (col)=3 ("disabled index (col)")) -> (element=w582:dbl)
            n107 = Index Array "array length"(array=w590) -> (element=w569:i32)  [unwired: 1 in]
            n108 = Index Array "time"(array=w568, index (row)=w562, index (col)=0) -> (element=w579:dbl)
            n109 = Greater Or Equal?(x=w569, y=w562) -> (x >= y?=w587:bool)
            n110 = Multiply(x=w579, y=60.0) -> (x*y=w567:dbl)
            n111 = call "Elapsed Time3"("Time Target (s)"=w567, "Auto Reset"=TRUE, "Set Start Time (s)"=w574) -> ("Elapsed Time (s)"=w566:dbl, "Time has Elapsed"=w586:bool)  [unwired: 9 in, 6 out]
            n112 = Increment(x=w562) -> (x+1=→"Current step":i32)
            n113 = Subtract(x=w567, y=w566) -> (x-y=w563:dbl)
            n114 = And(x=w586, y=w587) -> (x .and. y?=w559:bool)
            n115 = call "Elapsed Time4"("Reset"=FALSE, "Set Start Time (s)"=w574) -> ("Elapsed Time (s)"=w572:dbl)  [unwired: 10 in, 7 out]
            n116 = Increment(x=w562) -> (x+1=w576:i32)
            n117 = Divide(x=w563, y=60.0) -> (x/y=→"Step time remaining (min)":dbl)
            n118 = Select(t=w576, s=w559, f=w562) -> (s? t:f=w575:i32)
            n119 = Divide(x=w572, y=60.0) -> (x/y=w571:dbl)
          }
        }
        n120 = Index Array "vapor flow"(array=w512, index=4) -> (element=w508:dbl)
        n121 = Index Array "vacuum presure"(array=w512, index=0) -> ()  [unwired: 1 out]
        n122 = Index Array "high pressure"(array=w512, index=1) -> (element=w515:dbl)
        n123 = Index Array "low pressure"(array=w512, index=2) -> (element=w486:dbl)
        n124 = Index Array "gas flow"(array=w512, index=3) -> (element=w510:dbl)
        n125 = Greater Or Equal To 0?(x=w486) -> (x >= 0?=w487:bool)
        n126 = Multiply(x=40.0, y=w508) -> (x*y=w499:dbl)
        n127 = Multiply(x=40.0, y=w510) -> (x*y=w496:dbl)
        n128 = Greater Or Equal?(x=w496, y=1.0) -> (x >= y?=w495:bool)
        n129 = Select(t=w486, s=w487, f=0.0) -> (s? t:f=w485:dbl)
        n130 = Greater Or Equal?(x=w499, y=1.0) -> (x >= y?=w498:bool)
        n131 = Multiply(x=100.0, y=w515) -> (x*y=w503:dbl)
        n132 = Select(t=w496, s=w495, f=0.0) -> (s? t:f=w433:dbl)
        "Actual" <- w433
        n133 = Select(t=w499, s=w498, f=0.0) -> (s? t:f=w432:dbl)
        "Actual" <- w432
        n134 = Greater?(x=w485, y=10.0) -> (0:w491:bool)
        n135 = Greater Or Equal To 0?(x=w503) -> (x >= 0?=w505:bool)
        n136 = Select(t=w503, s=w505, f=0.0) -> (s? t:f=w490:dbl)
        n137 = Bundle("f"=w433, "f"=w432) -> (→"Waveform Chart 2":cluster{"f":dbl, "f":dbl})  [unwired: 1 in]
        n138 = Greater Than 0?(x=w433) -> (x > 0?=→"Boolean 3":bool)
        n139 = Select(t=w490, s=w491, f=w485) -> (s? t:f=w435:dbl)
        n140 = Greater Than 0?(x=w432) -> (x > 0?=→"Boolean":bool)
        n141 = Greater?(x=0.05, y=w435) -> (0:w456:bool)
        n142 = Bundle("f"=w435) -> (→"Chamber Pressure (Torr)":cluster{"f":dbl})  [unwired: 1 in]
        n143 = And(x=w456, y="Turbo pump auto on") -> (x .and. y?=w464:bool)
        n144 = Number To Engineering String(4:w433) -> (0:w481:string)  [unwired: 3 in]
        n145 = Number To Engineering String(4:w435) -> (0:w482:string)  [unwired: 3 in]
        n146 = Number To Engineering String(4:w432) -> (0:w479:string)  [unwired: 3 in]
        n147 = Build Array(w459, w458) -> (w457:dbl[])
        n148 = Subtract(x=w446, y=w445) -> (x-y=w428:dbl)
        n149 = Equal To 0?(x=w433) -> (x = 0?=w437:bool)
        n150 = Equal To 0?(x=w432) -> (x = 0?=w438:bool)
        n151 = Divide(x=w428, y=60.0) -> (x/y=→"Sequence time left (hrs)":dbl)
        n152 = And(x=w437, y=w438) -> (x .and. y?=w436:bool)
        n153 = case shown="False" w436 {
          tunnel: w435 -> [w536 w546]
          tunnel: [w535 w545] -> w434
          tunnel: w433 -> [w544 _]
          tunnel: w432 -> [w542 _]
          frame False {
            # "Calculate humidity when gas/vapor are flowing"
            n154 = Add(x=w544, y=w542) -> (x+y=w543:dbl)
            n155 = Divide(x=w542, y=w543) -> (x/y=w537:dbl)
            n156 = Multiply(x=w536, y=w537) -> (x*y=w538:dbl)
            n157 = Divide(x=w538, y=23.8) -> (x/y=w540:dbl)
            n158 = Multiply(x=w540, y=100.0) -> (x*y=w535:dbl)
          }
          frame True {
            # "calculate humidity when no gas/vapor are flowing"
            n159 = Divide(x=w546, y=23.8) -> (x/y=w548:dbl)
            n160 = Multiply(x=w548, y=100.0) -> (x*y=w545:dbl)
          }
        }
        n161 = Less Or Equal To 0?(x=w428) -> (x <= 0?=w421:bool)
        n162 = case "reinitialize \"run sequence\" button  when sequence ends" shown="True" w421 {
          tunnel: [TRUE ("Run Sequence") w551] -> w419
          frame False {
          }
          frame True {
            w551 = FALSE ("Run Sequence")
            n163 = property on="Run Sequence" class="Bool (strict)"("Value"=w551) -> ()  [unwired: 2 in, 2 out]
          }
        }
        n164 = call "butterfly_valve_subvi.vi"("Desired pressure"=w447, "error in (no error)"=w476, "Pressure Control"=w452, 10:"valve % open", "VISA Refnum in"=w475) -> ("error out"=w492:errorcluster, "Valve position (%)"=→"Valve position (%)":dbl, "VISA Refnum out"=w466:refnum<visa-resource-name>)  [unwired: 4 in]
        n165 = call-poly <vilib>:"DAQmx Write.vi"("task/channels in"=w470, "data"=w464, "error in"=w469) -> ("task out"=w468:refnum<k21>, "error out"=w467:errorcluster)  [unwired: 10 in, 1 out]
        n166 = Divide(x=w457, y=40.0 ("Waveform")) -> (x/y=w494:dbl[])
        n167 = call-poly <vilib>:"DAQmx Write.vi"("task/channels in"=w471, "data"=w494, "error in"=w472) -> ("task out"=w501:refnum<k21>, "error out"=w502:errorcluster)  [unwired: 10 in, 1 out]
        n168 = Number To Engineering String(4:w434) -> (0:w439:string)  [unwired: 3 in]
      }
    }
    n169 = case "Clear all graphs" shown="True" "Clear all charts" {
      frame False {
      }
      frame True {
        w606 = cluster{dbl, "Resistance out":dbl}[] [] ("History Data")
        w607 = cluster{dbl}[] [] ("History Data")
        n170 = property on="Keithley 2420 (Ohm)" class="WFChart (strict)"("History Data"=w607) -> ()  [unwired: 2 in, 2 out]
        n171 = property on="J-Kem Temp (C)" class="WFChart (strict)"("History Data"=w607) -> ()  [unwired: 2 in, 2 out]
        n172 = property on="Keithley 6430 (Ohm)" class="WFChart (strict)"("History Data"=w607) -> ()  [unwired: 2 in, 2 out]
        n173 = property on="Waveform Chart 7" class="WFChart (strict)"("History Data"=w606) -> ()  [unwired: 2 in, 2 out]
        n174 = property on="Waveform Chart" class="WFChart (strict)"("History Data"=w607) -> ()  [unwired: 2 in, 2 out]
        n175 = property on="Waveform Chart 6" class="WFChart (strict)"("History Data"=w607) -> ()  [unwired: 2 in, 2 out]
        n176 = property on="flow rates" class="WFChart (strict)"("History Data"=w606) -> ()  [unwired: 2 in, 2 out]
        n177 = property on="Chamber Pressure (Torr)" class="WFChart (strict)"("History Data"=w607) -> ()  [unwired: 2 in, 2 out]
        n178 = property on="Arduino humidity (%)" class="WFChart (strict)"("History Data"=w607) -> ()  [unwired: 2 in, 2 out]
        n179 = property on="Waveform Chart 8" class="WFChart (strict)"("History Data"=w606) -> ()  [unwired: 2 in, 2 out]
      }
    }
    n180 = Multiply(x=u32 1000, y="Delay between data points (s)") -> (x*y=w275:dbl)
    n181 = case "Setnag O2 Pump" shown="True" w288 {
      tunnel: [w686 w690] -> w303
      tunnel: w302 -> [w686 w691]
      tunnel: w275 -> [_ w687]
      tunnel: w294 -> [_ w689]
      tunnel: ["" w688] -> w293
      frame False {
      }
      frame True {
        # "SetNag O2 Gauge"
        n182 = flat-sequence {
          tunnel: [w700] -> w697
          tunnel: w687 -> [w702]
          tunnel: w689 -> [w700]
          tunnel: w697 -> [w703]
          tunnel: w687 -> [w710]
          tunnel: [w706] -> w690
          frame #0 {
            n183 = Wait (ms)(milliseconds to wait=w702) -> ()  [unwired: 1 out]
            n184 = call <vilib>:"Serial Port Write.vi"("string to write"="_OXY\r" ("O2 partial press"), "port number"=w700) -> ()  [unwired: 1 out]
          }
          frame #1 {
            # "O2 partial pressure"
            n185 = call <vilib>:"Bytes At Serial Port.vi"() -> ("byte count"=w711:u32)  [unwired: 1 in, 1 out]
            n186 = Wait (ms)(milliseconds to wait=w710) -> ()  [unwired: 1 out]
            n187 = call <vilib>:"Serial Port Read.vi"("requested byte count"=w711, "port number"=w703) -> ("string read"=w709:string)  [unwired: 1 out]
            n188 = Fract/Exp String To Number(string=w709) -> (number=w707:dbl)  [unwired: 3 in, 1 out]
            "atm" <- w707
            n189 = Multiply(x=w707, y=100.0) -> (x*y=w704:dbl)
            "%" <- w704
            n190 = Multiply(x=w704, y=7.6) -> (x*y=w706:dbl)
            "Torr" <- w706
          }
        }
        n191 = Wait (ms)(milliseconds to wait=w687) -> ()  [unwired: 1 out]
        n192 = Greater?(x=w690, y=1e-07) -> (0:w693:bool)
        n193 = case shown="False" w693 {
          tunnel: [w698 w699] -> w692
          tunnel: w690 -> [_ w699]
          tunnel: w691 -> [w698 _]
          frame False {
          }
          frame True {
          }
        }
        n194 = Number To Engineering String(4:w692) -> (0:w688:string)  [unwired: 3 in]
        n195 = Bundle(w688) -> (w695:cluster{string})  [unwired: 1 in]
        n196 = Fract/Exp String To Number(string=w695) -> (number=→"Waveform Chart":cluster{dbl})  [unwired: 3 in, 1 out]
      }
    }
    n197 = Equal To 0?(x=w229) -> (x = 0?=w219:bool)
    n198 = Wait (ms)(milliseconds to wait=w275) -> ()  [unwired: 1 out]
    n199 = case "SRS QCM" shown="True" w295 {
      selector: w295 -> [w659 w673]
      tunnel: w298 -> [w662 w677]
      tunnel: w297 -> [w661 w679]
      tunnel: [w657 w684] -> w296
      tunnel: [w657 w683] -> w292
      tunnel: [w660 w682] -> w289
      tunnel: w219 -> [_ w672]
      tunnel: w218 -> [_ w671]
      tunnel: [0.0 w668] -> w217
      tunnel: [w657 w666] -> w216
      frame False {
        w657 = ""
        n200 = Bundle(w659, "VISA out"=w662, "error out"=w661) -> (w660:T14)  [unwired: 1 in]
      }
      frame True {
        # "SRS QCM"
        n201 = call "Elapsed Time2"() -> ("Elapsed Time (s)"=w678:dbl)  [unwired: 12 in, 7 out]
        n202 = call "SrsQcm200FandR_MODIFIED.vi"("VISA in"=w677, "Reference time in"=w678, "error in (no error)"=w679) -> ("VISA out"=w675:refnum<visa-resource-name>, "Frequency out"=w667:dbl, "Resistance out"=w663:dbl, "error out"=w676:errorcluster)  [unwired: 6 in, 3 out]
        "Ohm" <- w663
        n203 = Select(t=w667, s=w672, f=w671) -> (s? t:f=w668:dbl)
        n204 = Bundle(w673, "VISA out"=w675, "error out"=w676) -> (w682:T14)  [unwired: 1 in]
        n205 = Number To Engineering String(4:w667) -> (0:w684:string)  [unwired: 3 in]
        n206 = Subtract(x=w668, y=w667) -> (x-y=w670:dbl)
        n207 = Divide(x=w667, y=1000000.0) -> (x/y=w674:dbl)
        "MHz" <- w674
        n208 = Number To Engineering String(4:w663) -> (0:w683:string)  [unwired: 3 in]
        n209 = Bundle(w674, "Resistance out"=w663) -> (→"Waveform Chart 7":cluster{dbl, "Resistance out":dbl})  [unwired: 1 in]
        n210 = Divide(x=w670, y=56.65) -> (x/y=w664:dbl)
        n211 = Bundle(w664, "Resistance out"=w663) -> (→"Waveform Chart 8":cluster{dbl, "Resistance out":dbl})  [unwired: 1 in]
        n212 = Number To Engineering String(4:w664) -> (0:w666:string)  [unwired: 3 in]
      }
    }
    n213 = case "Keithley 2420" shown="True" w272 {
      selector: w272 -> [w645 w653]
      tunnel: w300 -> [w644 w648]
      tunnel: w299 -> [w643 w647]
      tunnel: [w642 w651] -> w290
      tunnel: ["" w650] -> w291
      frame False {
        n214 = Bundle(w645, "VISA resource name out"=w644, "error out"=w643) -> (w642:T7)  [unwired: 1 in]
      }
      frame True {
        # "Keithley 2420"
        n215 = call-poly "Read.vi"("VISA resource name"=w648, "error in (no error)"=w647) -> ("VISA resource name out"=w654:refnum<visa-resource-name>, "Resistance"=w649:sgl, "error out"=w652:errorcluster)  [unwired: 7 in, 4 out]
        n216 = Bundle("Resistance"=w649) -> (→"Keithley 2420 (Ohm)":cluster{"Resistance":sgl})  [unwired: 1 in]
        n217 = Number To Engineering String(4:w649) -> (0:w650:string)  [unwired: 3 in]
        n218 = Wait (ms)(milliseconds to wait=u32 20) -> ()  [unwired: 1 out]
        n219 = Bundle(w653, "VISA resource name out"=w654, "error out"=w652) -> (w651:T7)  [unwired: 1 in]
      }
    }
    n220 = case "Keithley 6430" shown="True" w266 {
      selector: w266 -> [w594 w604]
      tunnel: w269 -> [w593 w601]
      tunnel: w268 -> [w592 w600]
      tunnel: ["" w603] -> w212
      tunnel: [w591 w602] -> w267
      frame False {
        n221 = Bundle(w594, "VISA resource name out"=w593, "error out"=w592) -> (w591:T7)  [unwired: 1 in]
      }
      frame True {
        # "Keithley 6430"
        n222 = call-poly "Read.vi"("error in (no error)"=w600, "VISA resource name"=w601) -> ("error out"=w599:errorcluster, "Measurement"=w597:dbl, "VISA resource name out"=w598:refnum<visa-resource-name>)  [unwired: 1 in, 6 out]
        n223 = Number To Engineering String(4:w597) -> (0:w603:string)  [unwired: 3 in]
        n224 = Bundle("Measurement"=w597) -> (→"Keithley 6430 (Ohm)":cluster{"Measurement":dbl})  [unwired: 1 in]
        n225 = Wait (ms)(milliseconds to wait=u32 20) -> ()  [unwired: 1 out]
        n226 = Bundle(w604, "VISA resource name out"=w598, "error out"=w599) -> (w602:T7)  [unwired: 1 in]
      }
    }
    n227 = Unbundle(w281) -> (w280:bool, "VISA resource name out"=w279:refnum<visa-resource-name>, "error out"=w278:errorcluster)
    n228 = call "J-KEM_subVI.vi"("Address in"=w287, "J-KEM on?"=w284) -> ("String data out"=w285:string, "plot data out"=→"J-Kem Temp (C)":cluster{"Numeric Control":dbl}, "Address out"=w286:T15)  [unwired: 7 in]
    n229 = Greater?(x=w229, y=1.0) -> (0:w236:bool)
    n230 = case "RapidOX O2 Sensor" shown="True" w280 {
      tunnel: w279 -> [_ w615]
      tunnel: w278 -> [w608 w614]
      tunnel: ["" w613] -> w277
      tunnel: [w608 w610] -> w276
      frame False {
      }
      frame True {
        # "RapidOX 2100"
        n231 = VISA Write(VISA resource name=w615, write buffer="D", error in (no error)=w614) -> (VISA resource name out=w618:refnum<visa-resource-name>, error out=w617:errorcluster)  [unwired: 1 out]
        n232 = flat-sequence {
          tunnel: [w627] -> w624
          tunnel: [w625] -> w623
          tunnel: w618 -> [w627]
          tunnel: w617 -> [w625]
          tunnel: w624 -> [w632]
          tunnel: w623 -> [w631]
          tunnel: [w630] -> w622
          tunnel: [w629] -> w621
          tunnel: [w628] -> w620
          tunnel: w622 -> [w641]
          tunnel: w621 -> [w640]
          tunnel: w620 -> [w639]
          tunnel: [w638] -> w610
          tunnel: [w633] -> w612
          frame #0 {
            n233 = Wait (ms)(milliseconds to wait=u32 100) -> ()  [unwired: 1 out]
          }
          frame #1 {
            n234 = property class="Instr"(reference=w632, error in=w631) -> (reference out=w630:refnum<visa-resource-name>, error out=w628:errorcluster, "Bytes at Port"=w629:u32)
          }
          frame #2 {
            n235 = VISA Read(VISA resource name=w641, byte count=w640, error in (no error)=w639) -> (read buffer=w636:string, error out=w638:errorcluster)  [unwired: 2 out]
            n236 = Match Pattern(string=w636, regular expression="d") -> (after substring=w634:string)  [unwired: 1 in, 3 out]
            n237 = Match Pattern(string=w634, regular expression=",") -> (before substring=w633:string)  [unwired: 1 in, 3 out]
          }
        }
        n238 = flat-sequence {
          frame #0 {
          }
        }
        n239 = Fract/Exp String To Number(string=w612) -> (number=w611:dbl)  [unwired: 3 in, 1 out]
        "O2 Concentration (PPM)" <- w611
        n240 = Bundle(w611) -> (→"Waveform Chart 6":cluster{dbl})  [unwired: 1 in]
        n241 = Number To Engineering String(4:w611) -> (0:w613:string)  [unwired: 3 in]
      }
    }
    n242 = And(x=w236, y=w237) -> (x .and. y?=w247:bool)
    n243 = case shown="True" w247 {
      selector: w247 -> [w373 w404]
      tunnel: w246 -> [w375 w383]
      tunnel: w245 -> [w374 w384]
      tunnel: [w375 w387] -> w243
      tunnel: [w374 w386] -> w242
      tunnel: [w373 w404] -> w244
      tunnel: [w372 w385] -> w241
      tunnel: [w372 w378] -> w238
      tunnel: [w372 w382] -> w239
      frame False {
        w372 = ""
      }
      frame True {
        n244 = property class="Instr"(reference=w383, error in=w384) -> (reference out=w401:refnum<visa-resource-name>, error out=w403:errorcluster, "Bytes at Port"=w402:u32)
        n245 = VISA Read(VISA resource name=w401, byte count=w402, error in (no error)=w403) -> (VISA resource name out=w387:refnum<visa-resource-name>, read buffer=w376:string, error out=w386:errorcluster)  [unwired: 1 out]
        n246 = flat-sequence {
          tunnel: [w406] -> w377
          tunnel: w376 -> [w406]
          frame #0 {
            n247 = Wait (ms)(milliseconds to wait=u32 1500) -> ()  [unwired: 1 out]
          }
        }
        n248 = Search/Split String(string=w377, search string/char (-)=":") -> (match + rest of string=w398:string)  [unwired: 1 in, 2 out]
        n249 = Search/Split String(string=w398, offset (0)=1) -> (match + rest of string=w396:string)  [unwired: 1 in, 2 out]
        n250 = Search/Split String(string=w396, search string/char (-)="h") -> (substring before match=w385:string, match + rest of string=w394:string)  [unwired: 1 in, 1 out]
        "gas\nsensor" <- w385
        n251 = Search/Split String(string=w394, offset (0)=2) -> (match + rest of string=w392:string)  [unwired: 1 in, 2 out]
        n252 = Search/Split String(string=w392, search string/char (-)="t") -> (substring before match=w382:string, match + rest of string=w390:string)  [unwired: 1 in, 1 out]
        n253 = Search/Split String(string=w390, offset (0)=2) -> (match + rest of string=w380:string)  [unwired: 1 in, 2 out]
        n254 = Fract/Exp String To Number(string=w382) -> (number=w388:dbl)  [unwired: 3 in, 1 out]
        n255 = Bundle(w388) -> (→"Arduino humidity (%)":cluster{dbl})  [unwired: 1 in]
        n256 = Search/Split String(string=w380, search string/char (-)=".", offset (0)=0) -> (substring before match=w378:string)  [unwired: 2 out]
        "temp\n(C)" <- w378
      }
    }
    n257 = Divide(x=w283, y=60.0) -> (x/y=w232:dbl)
    "Elapsed (min)" <- w232
    n258 = Multiply(x="hrs", y=60.0) -> (x*y=w226:dbl)
    n259 = Greater Or Equal?(x=w232, y="Start recording after") -> (x >= y?=w210:bool)
    n260 = Number To Engineering String "elapsed time (min)"(4:w232) -> (0:w304:string)  [unwired: 3 in]
    n261 = Greater Or Equal?(x=w232, y=w226) -> (x >= y?=w235:bool)
    n262 = And(x=w235, y="Auto stop after") -> (x .and. y?=w233:bool)
    n263 = Or(x="stop", y=w233) -> (x .or. y?=w213:bool)
    n264 = Get Date/Time In Seconds() -> (seconds since 1Jan1904=w305:timestamp)
    n265 = case shown="\"Save during sequence only\", Default" "Data saving" {
      tunnel: [w309 w314] -> w214
      tunnel: w213 -> [_ w314]
      tunnel: w211 -> [w310 _]
      tunnel: w210 -> [_ w313]
      tunnel: [w310 w313] -> w206
      tunnel: w208 -> [_ _]
      tunnel: "stop" -> [w308 _]
      tunnel: w207 -> [w306 _]
      frame "Save during sequence only", Default {
        w311 = T16."Disabled and Grayed Out" ("Disabled")
        n266 = property on="Start recording\nafter" class="DigNum (strict)"("DisabledEnum"=w311) -> ()  [unwired: 2 in, 2 out]
        n267 = property on="Auto stop after" class="Bool (strict)"("DisabledEnum"=w311) -> ()  [unwired: 2 in, 2 out]
        n268 = property on="hrs" class="DigNum (strict)"("DisabledEnum"=w311) -> ()  [unwired: 2 in, 2 out]
        n269 = Not(x=w306) -> (.not. x?=w307:bool)
        n270 = Or(x=w308, y=w307) -> (x .or. y?=w309:bool)
      }
      frame " Manually save data" {
        w312 = T16."Enabled" ("Disabled")
        n271 = property on="Start recording\nafter" class="DigNum (strict)"("DisabledEnum"=w312) -> ()  [unwired: 2 in, 2 out]
        n272 = property on="Auto stop after" class="Bool (strict)"("DisabledEnum"=w312) -> ()  [unwired: 2 in, 2 out]
        n273 = property on="hrs" class="DigNum (strict)"("DisabledEnum"=w312) -> ()  [unwired: 2 in, 2 out]
      }
    }
    "Currently saving data" <- w206
    n274 = Format Date/Time String(time format string (%c)="%Y-%m-%d %H:%M:%S%2u", seconds (now)=w305) -> (date/time string=w301:string)  [unwired: 1 in]
    n275 = Build Array(w301, w304, w212, w285, w291, w216, w296, w292, w293, w277, w259, w230, w258, w257, w241, w239, w238) -> (w240:string[])
  }
  n276 = Unbundle(w90) -> (w89:bool, "VISA out"=w88:refnum<visa-resource-name>, "error out"=w87:errorcluster)
  n277 = case shown="False" w89 {
    tunnel: w87 -> [w712 w715]
    tunnel: [w712 w714] -> w96
    tunnel: w88 -> [_ w713]
    frame False {
    }
    frame True {
      n278 = call "srsQcm200Close.vi"("error in"=w715, "Visa in"=w713) -> ("error out"=w714:errorcluster)  [unwired: 3 in]
    }
  }
  n279 = Unbundle(w85) -> ("Boolean"=w84:bool, "VISA resource name out"=w83:refnum<visa-resource-name>, "error out"=w82:errorcluster)
  n280 = Unbundle(w94) -> (w93:bool, "VISA resource name out"=w92:refnum<visa-resource-name>, "error out"=w91:errorcluster)
  n281 = case shown="True" w33 {
    tunnel: w32 -> [_ w717]
    tunnel: w31 -> [_ w718]
    frame False {
    }
    frame True {
      n282 = VISA Close(VISA resource name=w717, error in (no error)=w718) -> ()  [unwired: 1 out]
      n283 = call <vilib>:"Close.vi"("Arduino Resource"=T17 {"VISA resource"="", "Board Type"=enum."Uno", "Connection Type"=enum."USB / Serial", "Bytes Per Packet (15)"=15}) -> ()  [unwired: 14 in, 1 out]
    }
  }
  n284 = Unbundle(w57) -> (w62:bool, "VISA resource name out"=w61:refnum<visa-resource-name>, "error out"=w60:errorcluster)
  n285 = case shown="True" w49 {
    tunnel: [w719 w739] -> w47
    tunnel: w50 -> [_ w738]
    tunnel: w51 -> [_ w737]
    tunnel: w53 -> [_ w733]
    tunnel: w52 -> [_ w732]
    tunnel: [w719 w731] -> w48
    tunnel: [w720 w728] -> w46
    tunnel: w45 -> [w720 w727]
    tunnel: w37 -> [_ w724]
    tunnel: [w719 w723] -> w40
    tunnel: w39 -> [_ w722]
    tunnel: w38 -> [_ w721]
    frame False {
      w719 = errorcluster {"status"=FALSE, "code"=0, "source"=""} ("error out")
    }
    frame True {
      n286 = call <vilib>:"DAQmx Stop Task.vi"("task/channels in"=w722, "error in"=w721) -> ("task out"=w725:refnum<k21>, "error out"=w726:errorcluster)  [unwired: 12 in]
      n287 = call <vilib>:"DAQmx Stop Task.vi"("task/channels in"=w733, "error in"=w732) -> ("task out"=w735:refnum<k21>, "error out"=w734:errorcluster)  [unwired: 12 in]
      n288 = call <vilib>:"DAQmx Stop Task.vi"("task/channels in"=w738, "error in"=w737) -> ("task out"=w736:refnum<k21>, "error out"=w740:errorcluster)  [unwired: 12 in]
      n289 = VISA Clear(VISA resource name=w724, error in (no error)=w727) -> (VISA resource name out=w730:refnum<visa-resource-name>, error out=w729:errorcluster)
      n290 = call <vilib>:"DAQmx Clear Task.vi"("task in"=w725, "error in"=w726) -> ("error out"=w723:errorcluster)  [unwired: 13 in]
      n291 = call <vilib>:"DAQmx Clear Task.vi"("task in"=w735, "error in"=w734) -> ("error out"=w731:errorcluster)  [unwired: 13 in]
      n292 = call <vilib>:"DAQmx Clear Task.vi"("task in"=w736, "error in"=w740) -> ("error out"=w739:errorcluster)  [unwired: 13 in]
      n293 = VISA Close(VISA resource name=w730, error in (no error)=w729) -> (error out=w728:errorcluster)
    }
  }
  n294 = case shown="True" w93 {
    tunnel: w92 -> [_ w744]
    tunnel: w91 -> [w741 w743]
    tunnel: [w741 w742] -> w95
    frame False {
    }
    frame True {
      n295 = call "Enable Output.vi"("error in (no error)"=w743, "Enable Output (T: Enable)"=FALSE, "VISA resource name"=w744) -> ("error out"=w745:errorcluster, "VISA resource name out"=w747:refnum<visa-resource-name>)  [unwired: 7 in]
      n296 = call <vilib>:"Close.vi"("error in (no error)"=w745, "VISA resource name"=w747) -> ("error out"=w742:errorcluster)  [unwired: 9 in]
    }
  }
  n297 = case shown="True" w62 {
    tunnel: w61 -> [_ w750]
    tunnel: w60 -> [w748 w749]
    tunnel: [w748 w751] -> w56
    frame False {
    }
    frame True {
      w754 = FALSE  # Output (F:Off)
      n298 = call "Enable Output.vi"("error in (no error)"=w749, "Enable Output (F:Off)"=w754, "VISA resource name"=w750) -> ("error out"=w752:errorcluster, "VISA resource name out"=w753:refnum<visa-resource-name>)  [unwired: 7 out]
      n299 = call <vilib>:"Close.vi"("error in (no error)"=w752, "VISA resource name"=w753) -> ("error out"=w751:errorcluster)  [unwired: 9 out]
    }
  }
  n300 = case shown="True" w84 {
    tunnel: w83 -> [_ w758]
    tunnel: w82 -> [w755 w757]
    tunnel: [w755 w756] -> w81
    frame False {
    }
    frame True {
      n301 = VISA Close(VISA resource name=w758, error in (no error)=w757) -> (error out=w756:errorcluster)
    }
  }
  n302 = Merge Errors(w40, w48, w47, w46) -> (w18:errorcluster)
  n303 = Merge Errors(w17, w18) -> (w19:errorcluster)
  n304 = call <vilib>:"Simple Error Handler.vi"("error in (no error)"=w19) -> ()  [unwired: 4 in, 5 out]
  n305 = Merge Errors(w56, w81, w95, w96) -> (w103:errorcluster)
  n306 = call <vilib>:"Simple Error Handler.vi"("error in (no error)"=w103) -> ()  [unwired: 4 in, 5 out]
  n307 = Build Array("date/time", "min elapsed", "Keithley 6430 R (Ohm)", "J-KEM temp (C)", "Keithley 2420 R (Ohm)" ("element"), "QCM mass (ug)", "QCM f (Hz)", "QCM R (Ohm)", "O2 PP (Torr)" ("element"), "O2 conc (PPM)" ("element"), "pressure (Torr)" ("element"), "RH (%)" ("element"), "gas flow (sccm)" ("element"), "vapor flow (sccm)" ("element"), "gas sensor" ("element"), "humidity (%)" ("element"), "temp (C)" ("element"), "Experiment Notes") -> (w73:string[])
  n308 = call-poly <vilib>:"Write To Spreadsheet File.vi"("1D data"=w73, "file path (dialog if empty)"=w66) -> ("new file path (Not A Path if cancelled)"=w74:path)  [unwired: 6 in]
  n309 = call-poly <vilib>:"Write To Spreadsheet File.vi"("append to file? (new file:F)"=TRUE, "2D data"=w102, "file path (dialog if empty)"=w74) -> ()  [unwired: 5 in, 1 out]
